vi "macro_BoolCmd_RecvMultiplexerArray.vi"() -> ()   [LabVIEW 2019, in "Trajectory_Library.lvlib"]
uses:
  VI/BoolCmd_Recv_Internal.vi
  VI/DigSeqLogic_Edge_On.vi
  VI/BoolCmd_ObtainQueue.vi
  Trajectory_Library.lvlib
panel:
  out "Do Command 6":bool
  out "Do Command 5":bool
  out "Do Command 4":bool
  out "Do Command 3":bool
  in  "Ready6":bool=TRUE
  in  "Ready5":bool=TRUE
  in  "Ready4":bool=TRUE
  in  "Ready3":bool=TRUE
  in  "Ready2":bool=TRUE
  out "Do Cancel":bool
  out "Do Command 2":bool
  out "Do Command 1":bool
  in  "Ready1":bool=TRUE
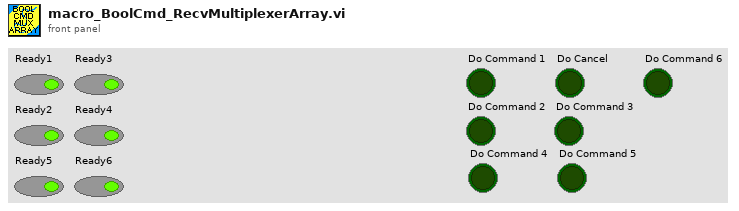
[diagram p1: front panel]
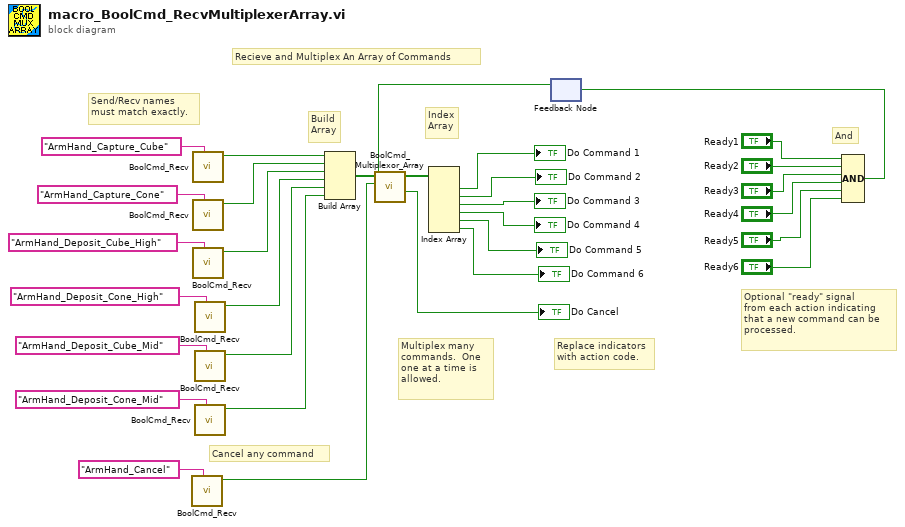
[diagram p0: block diagram]
diagram:
  # "And"
  # "Cancel any command"
  # "Index\nArray"
  # "Build\nArray"
  # "Replace indicators\nwith action code."
  # "Optional \"ready\" signal\nfrom each action indicating\nthat a new command can be\nprocessed."
  # "Multiplex many\ncommands.  One\none at a time is \nallowed."
  # "Send/Recv names\nmust match exactly."
  # "Recieve and Multiplex An Array of Commands"
  n1 = call "BoolCmd_Recv.vi"("Command Name"="ArmHand_Cancel") -> ("New Request"=w28:bool)  [unwired: 9 in, 1 out]
  n2 = call "BoolCmd_Recv.vi"("Command Name"="ArmHand_Capture_Cube") -> ("New Request"=w21:bool)  [unwired: 9 in, 1 out]
  n3 = call "BoolCmd_Recv.vi"("Command Name"="ArmHand_Capture_Cone") -> ("New Request"=w20:bool)  [unwired: 9 in, 1 out]
  n4 = call "BoolCmd_Recv.vi"("Command Name"="ArmHand_Deposit_Cube_High") -> ("New Request"=w12:bool)  [unwired: 9 in, 1 out]
  n5 = call "BoolCmd_Recv.vi"("Command Name"="ArmHand_Deposit_Cone_High") -> ("New Request"=w11:bool)  [unwired: 9 in, 1 out]
  n6 = call "BoolCmd_Recv.vi"("Command Name"="ArmHand_Deposit_Cube_Mid") -> ("New Request"=w10:bool)  [unwired: 9 in, 1 out]
  n7 = call "BoolCmd_Recv.vi"("Command Name"="ArmHand_Deposit_Cone_Mid") -> ("New Request"=w9:bool)  [unwired: 9 in, 1 out]
  n8 = Build Array(w21, w20, w12, w11, w10, w9) -> (w22:bool[])
  n9 = feedback #1() -> (w23:bool)  [unwired: 1 in]
  n10 = call "BoolCmd_Multiplexor_Array.vi"("Ready"=w23, "Command Cancel"=w28, "Commands"=w22) -> ("Do Cancel"=→"Do Cancel":bool, "Do Command"=w19:bool[])  [unwired: 7 in]
  n11 = Index Array(array=w19) -> (element #1=→"Do Command 1":bool, element #2=→"Do Command 2":bool, element #3=→"Do Command 3":bool, element #4=→"Do Command 4":bool, element #5=→"Do Command 5":bool, element #6=→"Do Command 6":bool)  [unwired: 6 in]
  n12 = Compound Arithmetic op=AND("Ready1", "Ready2", "Ready3", "Ready4", "Ready5", "Ready6") -> (w24:bool)
  n13 = feedback-in #1(w24) -> ()
